vi "SetupInterface.vi"(8 "error in (no error)":errorcluster, 11 "AbstractStep in":refnum<class "Move.lvclass">) -> (0 "error out":errorcluster, 3 "AbstractStep out":refnum<class "Move.lvclass">)   [LabVIEW 2014, in "Move.lvclass"]
uses:
  Move.lvclass
  StepData/Control/MoveData.ctl
  StepData/StepData.lvclass
panel:
  in  "Sensor 4":bool
  in  "Sensor 3":bool
  in  "Sensor 2":bool
  in  "Sensor 1":bool
  in  "Mode":u16(ring) items=["Abs"=2, "Inc"=3]
  in  "Axis":u16(ring)=1 items=["X"=1, "Y"=2, "Z"=3, "Rotation"=4]
  in  "Position":dbl format="%#.2f"
  in  "Acc/Dec":dbl
  in  "Speed":dbl
  out "Step Name":string
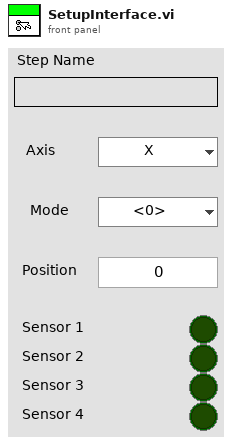
[diagram p1: front panel]
types:
  T1 = typedef "StepData.lvclass/MoveData.ctl" = cluster{"Axis":u16, "Position":dbl, "Speed":dbl, "Acc/Dec":dbl, "Mode":u16}
  T2 = typedef "StepData.lvclass/AllStepTypeData.ctl" = cluster{"StepName":string, "StepTypeEnum":T3, "MoveData":T1, "MeasureData":T4}
  T3 = typedef "StepData.lvclass/StepTypeEnum.ctl" = enum16{"Move", "Measure"}
  T4 = typedef "StepData.lvclass/MeasureData.ctl" = cluster{"Sensor No.":i32, "Log?":bool}
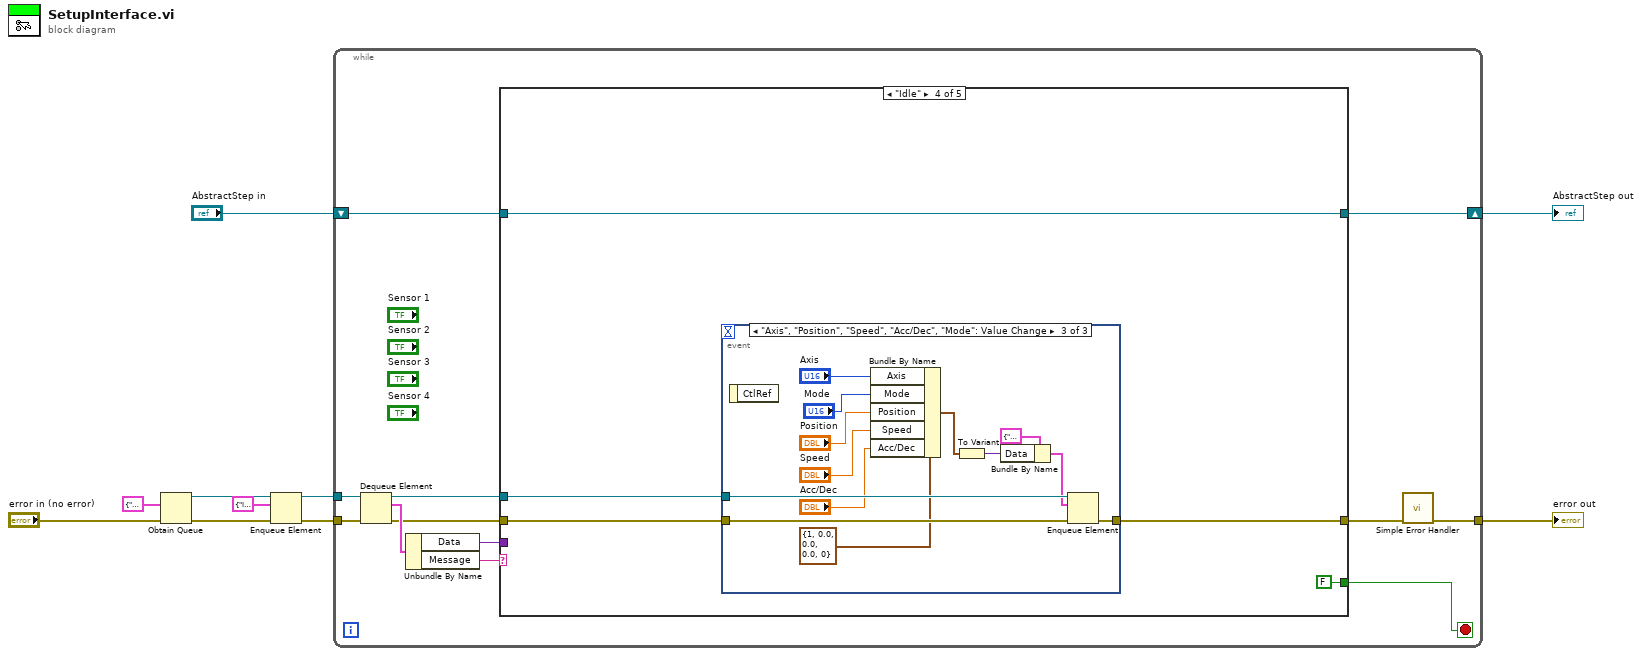
[diagram p0: block diagram]
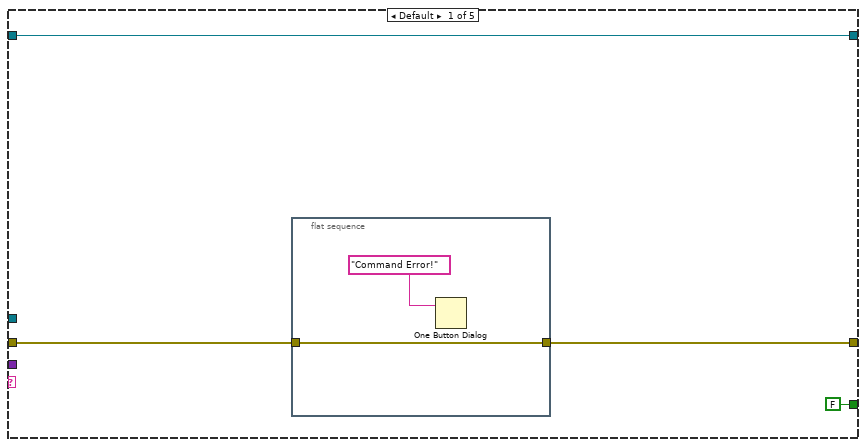
[diagram p2: hidden frame]
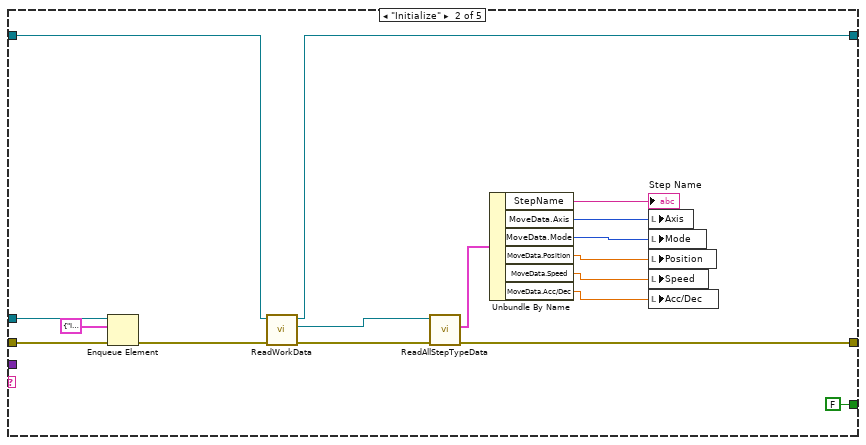
[diagram p3: hidden frame]
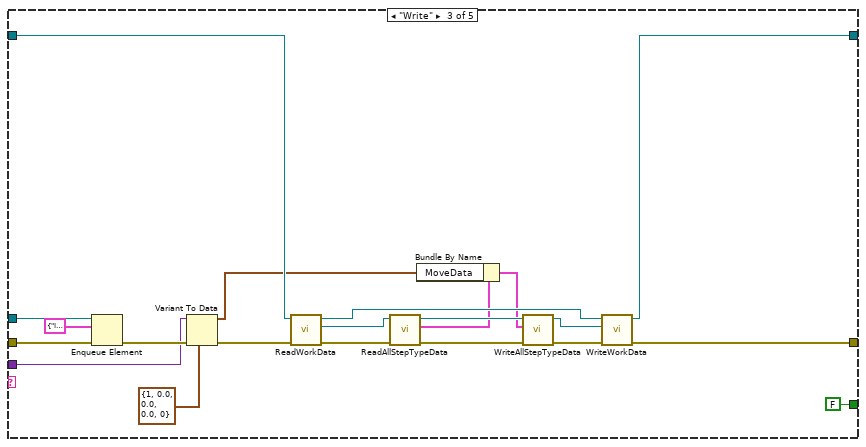
[diagram p4: hidden frame]
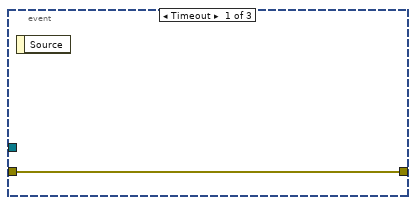
[diagram p5: hidden frame]
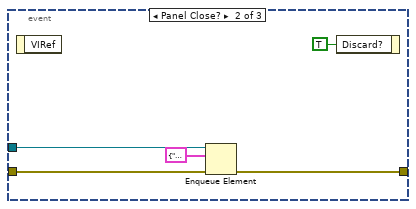
[diagram p6: hidden frame]
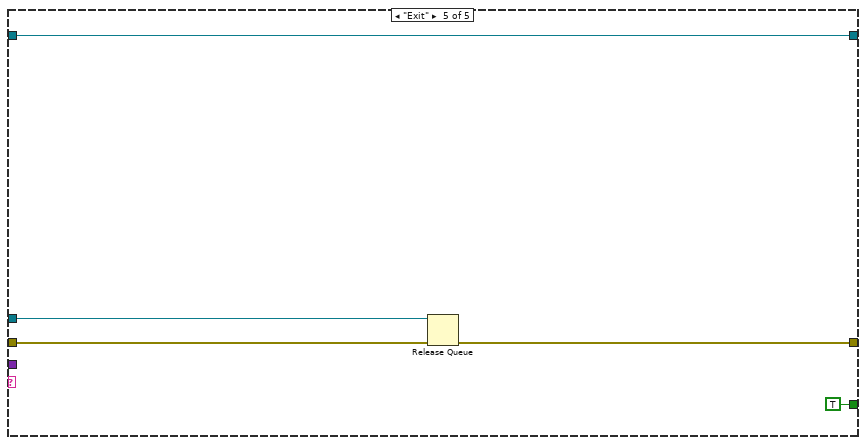
[diagram p7: hidden frame]
diagram:
  n1 = Obtain Queue(element data type=cluster{"Message":string, "Data":variant} {"Message"="", "Data"=variant}, error in (no error)="error in (no error)") -> (queue out=w9:refnum<queue>, error out=w10:errorcluster)  [unwired: 3 in, 1 out]
  n2 = Enqueue Element(queue=w9, element=cluster{"Message":string, "Data":variant} {"Message"="Initialize", "Data"=variant}, error in (no error)=w10) -> (queue out=w6:refnum<queue>, error out=w5:errorcluster)  [unwired: 1 in, 1 out]
  n3 = while {
    tunnel: w6 -> [w22]
    tunnel: w5 -> [w21]
    tunnel: [w14] -> w3
    shift-right: [w12] -> w1
    shift-left: "AbstractStep in" -> [w13]
    stop <- w15 stop-if-true
    n4 = Dequeue Element(queue=w22, error in (no error)=w21) -> (queue out=w16:refnum<queue>, element=w20:cluster{"Message":string, "Data":variant}, error out=w18:errorcluster)  [unwired: 1 in, 1 out]
    n5 = Unbundle By Name(w20) -> ("Data"=w11:variant, "Message"=w19:string)
    n6 = case shown="\"Idle\"" w19 {
      tunnel: w18 -> [w26 w45 w66 w70 w94]
      tunnel: [w25 w36 w55 w69 w92] -> w17
      tunnel: w16 -> [_ w44 w65 w71 w93]
      tunnel: [FALSE FALSE FALSE FALSE TRUE] -> w15
      tunnel: w13 -> [w23 w39 w61 w67 w91]
      tunnel: [w23 w40 w53 w67 w91] -> w12
      tunnel: w11 -> [_ _ w49 _ _]
      frame Default {
        n7 = flat-sequence {
          tunnel: w26 -> [w28]
          tunnel: [w28] -> w25
          frame #0 {
            n8 = One Button Dialog(message="Command Error!") -> ()  [unwired: 1 in, 1 out]
          }
        }
      }
      frame "Initialize" {
        n9 = Enqueue Element(queue=w44, element=cluster{"Message":string, "Data":variant} {"Message"="Idle", "Data"=variant}, error in (no error)=w45) -> (error out=w41:errorcluster)  [unwired: 1 in, 2 out]
        n10 = call-dynamic "ReadWorkData.vi"("error in (no error)"=w41, "AbstractStep in"=w39) -> ("error out"=w37:errorcluster, "StepData.lvclass"=w38:refnum<class "StepData.lvclass">, "AbstractStep out"=w40:refnum<class "Move.lvclass">)  [unwired: 7 in]
        n11 = call "ReadAllStepTypeData.vi"("error in (no error)"=w37, "StepData.lvclass In"=w38) -> ("error out"=w36:errorcluster, "AllStepTypeData"=w35:T2)  [unwired: 7 in, 1 out]
        n12 = Unbundle By Name(w35) -> ("StepName"=→"Step Name":string, "MoveData.Axis"=w33:u16, "MoveData.Mode"=w29:u16, "MoveData.Position"=w32:dbl, "MoveData.Speed"=w30:dbl, "MoveData.Acc/Dec"=w31:dbl)
        n13 = local write "Axis"(w33) -> ()
        n14 = local write "Mode"(w29) -> ()
        n15 = local write "Position"(w32) -> ()
        n16 = local write "Speed"(w30) -> ()
        n17 = local write "Acc/Dec"(w31) -> ()
      }
      frame "Write" {
        n18 = Enqueue Element(queue=w65, element=cluster{"Message":string, "Data":variant} {"Message"="Idle", "Data"=variant}, error in (no error)=w66) -> (error out=w50:errorcluster)  [unwired: 1 in, 2 out]
        n19 = Variant To Data(error in=w50, type=T1 {"Axis"=1, "Position"=0.0, "Speed"=0.0, "Acc/Dec"=0.0, "Mode"=0} ("MoveData"), Variant=w49) -> (data=w47:T1, error out=w46:errorcluster)
        n20 = call-dynamic "ReadWorkData.vi"("error in (no error)"=w46, "AbstractStep in"=w61) -> ("error out"=w62:errorcluster, "StepData.lvclass"=w60:refnum<class "StepData.lvclass">, "AbstractStep out"=w56:refnum<class "Move.lvclass">)  [unwired: 7 in]
        n21 = call "ReadAllStepTypeData.vi"("error in (no error)"=w62, "StepData.lvclass In"=w60) -> ("error out"=w58:errorcluster, "AllStepTypeData"=w52:T2, "StepData.lvclass Out"=w59:refnum<class "StepData.lvclass">)  [unwired: 7 in]
        n22 = Bundle By Name(cluster=w52, "MoveData"=w47) -> (w51:T2)
        n23 = call "WriteAllStepTypeData.vi"("error in (no error)"=w58, "AllStepTypeData"=w51, "StepData.lvclass In"=w59) -> ("error out"=w54:errorcluster, "StepData.lvclass Out"=w57:refnum<class "StepData.lvclass">)  [unwired: 7 in]
        n24 = call-dynamic "WriteWorkData.vi"("error in (no error)"=w54, "StepData.lvclass"=w57, "AbstractStep in"=w56) -> ("error out"=w55:errorcluster, "AbstractStep out"=w53:refnum<class "Move.lvclass">)  [unwired: 7 in]
      }
      frame "Idle" {
        n25 = event shown="[2] \"Axis\", \"Position\", \"Speed\", \"Acc/Dec\", \"Mode\": Value Change" {
          selector: _ -> [_ _ _]
          dyn-events: _ -> [_ _ _]
          timeout: _ -> [_ _ _]
          tunnel: w71 -> [_ w74 w88]
          tunnel: w70 -> [w72 w76 w90]
          tunnel: [w72 w75 w89] -> w69
          event Timeout {
            n26 = event-data() -> ()  [unwired: 1 in, 1 out]
          }
          event Panel Close? {
            n27 = event-data() -> ()  [unwired: 1 in, 1 out]
            n28 = Enqueue Element(queue=w74, element=cluster{"Message":string, "Data":variant} {"Message"="Exit", "Data"=variant}, error in (no error)=w76) -> (error out=w75:errorcluster)  [unwired: 1 in, 2 out]
            n29 = event-data("Discard?"=TRUE) -> ()  [unwired: 1 in, 1 out]
          }
          event "Axis", "Position", "Speed", "Acc/Dec", "Mode": Value Change {
            n30 = event-data() -> ()  [unwired: 1 in, 1 out]
            n31 = Bundle By Name(cluster=T1 {"Axis"=1, "Position"=0.0, "Speed"=0.0, "Acc/Dec"=0.0, "Mode"=0} ("MoveData"), "Axis"="Axis", "Mode"="Mode", "Position"="Position", "Speed"="Speed", "Acc/Dec"="Acc/Dec") -> (w84:T1)
            n32 = To Variant(anything=w84) -> (Variant=w86:variant)
            n33 = Bundle By Name(cluster=cluster{"Message":string, "Data":variant} {"Message"="Write", "Data"=variant} ("element"), "Data"=w86) -> (w81:cluster{"Message":string, "Data":variant})
            n34 = Enqueue Element(queue=w88, element=w81, error in (no error)=w90) -> (error out=w89:errorcluster)  [unwired: 1 in, 2 out]
          }
        }
      }
      frame "Exit" {
        n35 = Release Queue(queue=w93, error in (no error)=w94) -> (error out=w92:errorcluster)  [unwired: 1 in, 2 out]
      }
    }
    n36 = call <vilib>:"Simple Error Handler.vi"("error in (no error)"=w17) -> ("error out"=w14:errorcluster)  [unwired: 4 in, 4 out]
  }
  "error out" <- w3
  "AbstractStep out" <- w1
